vi "test_Checksum U8 - Check Protection with corrupt data.vi"(8 "error in (no error)":errorcluster) -> (0 "error out":errorcluster)   [LabVIEW 2023, in "Instrument Addon Protections Unit Tests.lvclass"]
uses:
  Instrument Addon Protections Unit Tests.lvclass
  <vilib>/addons/_JKI Toolkits/VI Tester/TestCase.llb/TestCase.lvclass
  Checksum U8/Checksum U8.lvclass
panel:
  out "Checksum U8 out":refnum<class "Checksum U8.lvclass">
  in  "Checksum U8 in":refnum<class "Checksum U8.lvclass">
  out "TestCase out":refnum<class "Instrument Addon Protections Unit Tests.lvclass">
  in  "TestCase in":refnum<class "Instrument Addon Protections Unit Tests.lvclass">
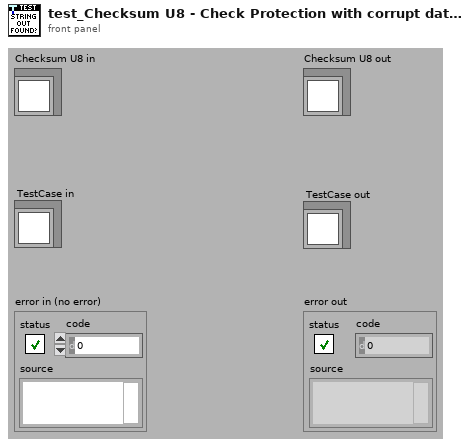
[diagram p1: front panel]
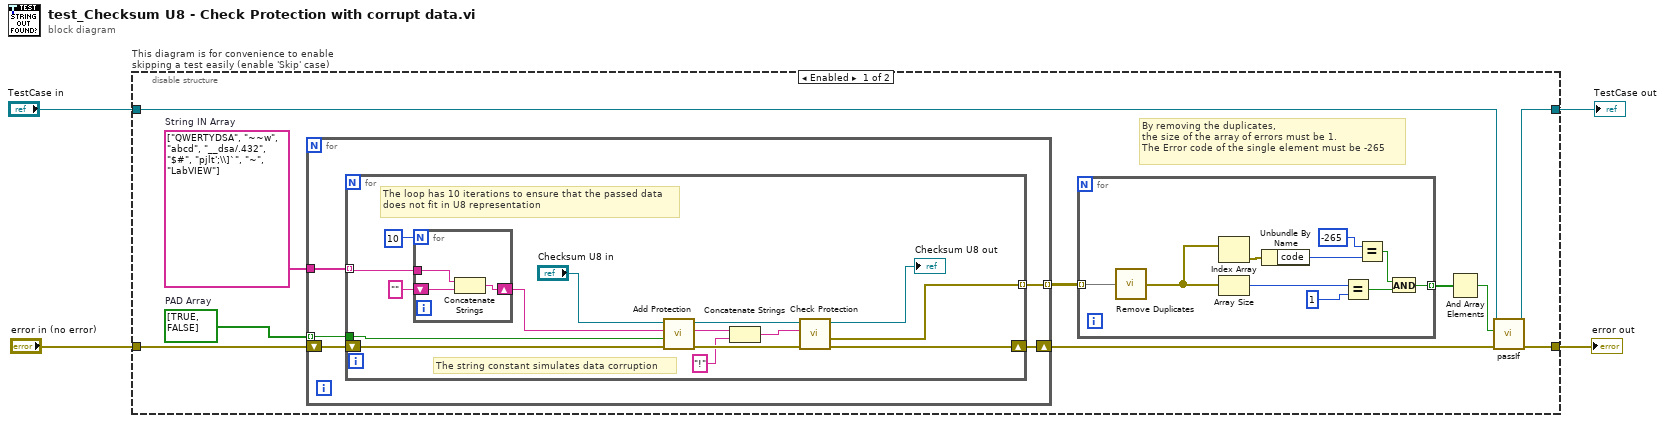
[diagram p0: block diagram]
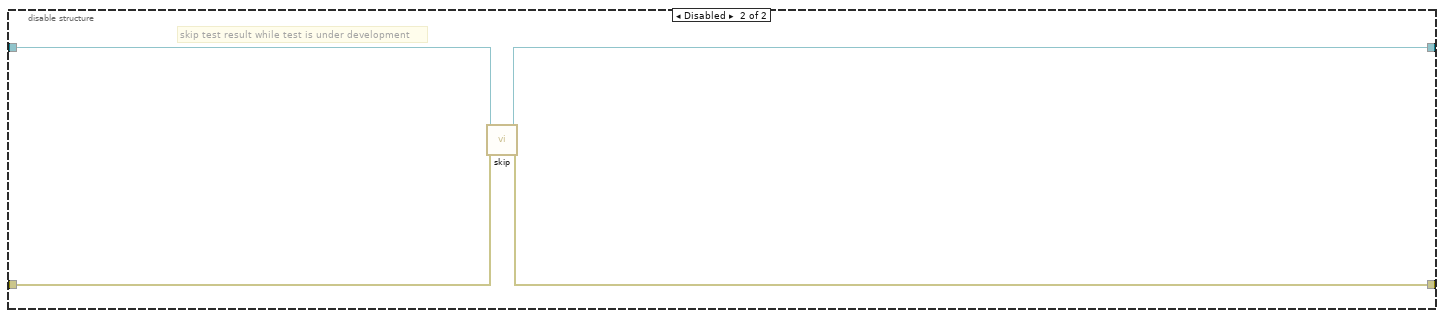
[diagram p2: hidden frame]
diagram:
  n1 = disable-structure "This diagram is for convenience to enable skipping a test easily (enable 'Skip' case)" shown="Enabled" {
    disable-tunnel: "TestCase in" -> [w12 w51]
    disable-tunnel: [w11 w49] -> w1
    disable-tunnel: [w10 w50] -> w3
    disable-tunnel: "error in (no error)" -> [w14 w48]
    frame Enabled {
      w7 = bool[] [TRUE, FALSE]  # PAD Array
      w13 = string[] ["QWERTYDSA", "~~w", "abcd", "__dsa/.432", "$#", "pjlt';\\]`", "~", "LabVIEW"]  # String IN Array
      # "By removing the duplicates, \nthe size of the array of errors must be 1. \nThe Error code of the single element must be -265"
      n2 = for {
        tunnel: w13 -> [w28]
        tunnel: [w26] -> w8 mode=indexing
        shift-right: [w27] -> w9
        shift-left: w14 -> [w29]
        tunnel: w7 -> [w25] mode=indexing
        n3 = for {
          tunnel: w28 -> [w42] mode=indexing
          shift-right: [w32] -> w27
          shift-left: w29 -> [w41]
          tunnel: [w31] -> w26 mode=indexing
          tunnel: w25 -> [w30]
          # "The string constant simulates data corruption"
          # "The loop has 10 iterations to ensure that the passed data\ndoes not fit in U8 representation"
          n4 = for {
            N: 10 -> [_]
            shift-right: [w47] -> w40
            shift-left: "" -> [w46]
            tunnel: w42 -> [w45]
            n5 = Concatenate Strings(w45, w46) -> (w47:string)
          }
          n6 = call-dynamic "Add Protection.vi"("error in (no error)"=w41, "Pad"=w30, "String in"=w40, "Checksum U8 in"="Checksum U8 in") -> ("error out"=w36:errorcluster, "String out"=w35:string, "Checksum U8 out"=w38:refnum<class "Checksum U8.lvclass">)  [unwired: 5 in]
          n7 = Concatenate Strings(w35, "!" ("string")) -> (w34:string)
          n8 = call-dynamic "Check Protection.vi"("error in (no error)"=w36, "String in"=w34, "Checksum U8 in"=w38) -> ("error out"=w32:errorcluster, "Protection Error"=w31:errorcluster, "Checksum U8 out"=→"Checksum U8 out":refnum<class "Checksum U8.lvclass">)  [unwired: 5 in, 1 out]
        }
      }
      n9 = for {
        tunnel: w8 -> [w16] mode=indexing
        tunnel: [w21] -> w6 mode=indexing
        n10 = call "Remove Duplicates.vi"("Array In"=w16) -> ("Array Out"=w15:errorcluster[])
        n11 = Index Array(array=w15) -> (element=w18:errorcluster)  [unwired: 1 in]
        n12 = Array Size(array=w15) -> (size(s)=w17:i32)
        n13 = Unbundle By Name(w18) -> ("code"=w19:i32)
        n14 = Equal?(x=w17, y=1) -> (x = y?=w22:bool)
        n15 = Equal?(x=-265, y=w19) -> (x = y?=w23:bool)
        n16 = And(x=w23, y=w22) -> (x .and. y?=w21:bool)
      }
      n17 = And Array Elements(Boolean array=w6) -> (logical AND=w5:bool)
      n18 = call-dynamic "passIf.vi"("error in (no error)"=w9, "pass"=w5, "TestCase in"=w12) -> ("error out"=w10:errorcluster, "TestCase out"=w11:refnum<class "Instrument Addon Protections Unit Tests.lvclass">)  [unwired: 7 in]
    }
    frame Disabled {
      # "skip test result while test is under development"
      n19 = call <vilib>:"skip.vi"("error in (no error)"=w48, "TestCase in"=w51) -> ("error out"=w50:errorcluster, "TestCase out"=w49:refnum<class "Instrument Addon Protections Unit Tests.lvclass">)  [unwired: 8 in]
    }
  }
  "error out" <- w3
  "TestCase out" <- w1
